vi "Filter Tree Edit Cell Event.vi"(8 "error in (no error)":errorcluster, 10 "TreeEditCellMsg":refnum<class "TreeEditCellMsg.lvclass">, 11 "IEventFilter in":refnum<class "IEventFilter.lvclass">) -> (0 "error out":errorcluster, 1 "Discard?":bool, 2 "Filtered String":string, 3 "IEventFilter out":refnum<class "IEventFilter.lvclass">, 5 "Data Filtered?":bool)   [LabVIEW 2020, in "MVA Framework.lvlib" / "ActorEvents.lvlib" / "IEventFilter.lvclass"]
doc: "过滤树形编辑单元格事件"
uses:
  IEventFilter.lvclass
  IEventAggregator Messages/TreeEditCellMsg/TreeEditCellMsg.lvclass
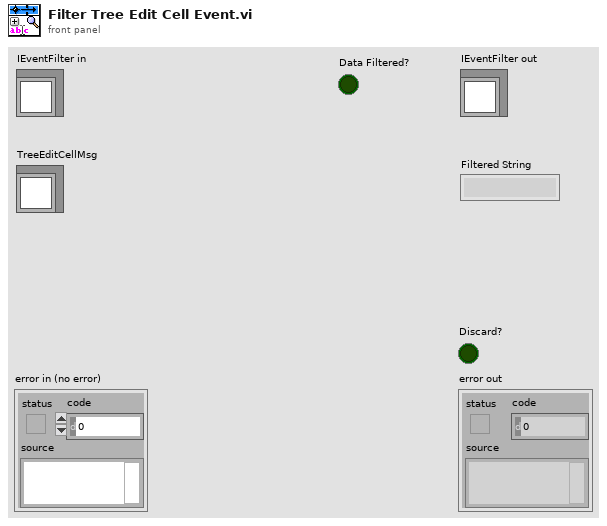
[diagram p1: front panel]
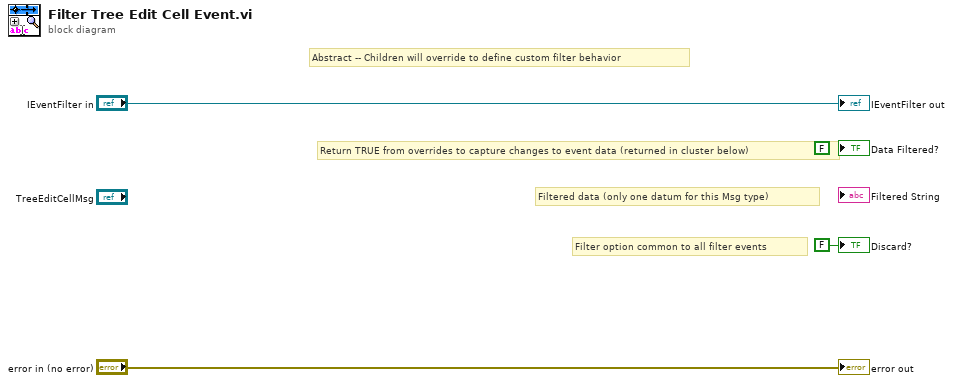
[diagram p0: block diagram]
diagram:
  # "Filtered data (only one datum for this Msg type)"
  # "Filter option common to all filter events"
  # "Return TRUE from overrides to capture changes to event data (returned in cluster below)"
  # "Abstract -- Children will override to define custom filter behavior"
  "error out" <- "error in (no error)"
  "IEventFilter out" <- "IEventFilter in"
  "Discard?" <- FALSE ("Discard?")
  "Data Filtered?" <- FALSE ("Data Filtered?")
